vi "Eliminated.vi"(6 "Column":i32, 8 "Row":i32, 9 "Killer":i32, 10 "Team":i32, 11 "Uno in":refnum<class "Uno.lvclass">) -> (3 "Uno out":refnum<class "Uno.lvclass">)   [LabVIEW 2017, in "Uno.lvclass"]
uses:
  Uno.lvclass
  Square/Square.lvclass
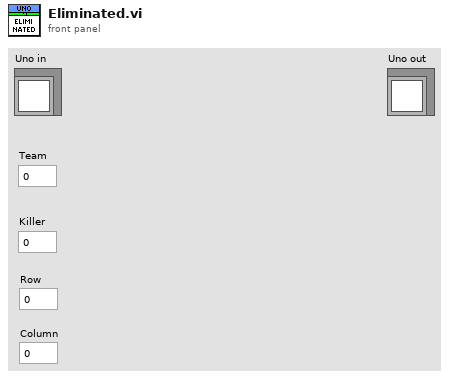
[diagram p1: front panel]
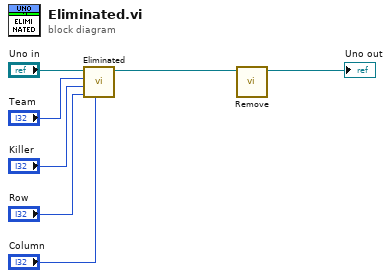
[diagram p0: block diagram]
diagram:
  n1 = call-parent "Eliminated.vi"("Column"="Column", "Row"="Row", "Killer Index"="Killer", "Team Index"="Team", "Square in"="Uno in") -> ("Square out"=w2:refnum<class "Uno.lvclass">)  [unwired: 6 in]
  n2 = call "Remove.vi"("Uno in"=w2) -> ("Uno out"=→"Uno out":refnum<class "Uno.lvclass">)  [unwired: 9 in, 1 out]
